vi "VI Tree.vi"   [LabVIEW 2015, in "IT-M3400.lvlib"]
doc: "This is the instrument driver for the <INSTRUMENT NAME>. The VI Tree displays all the user-callable VIs of the instrument driver in an organized table."
uses:
  <instrlib>/IT-M3400/IT-M3400.lvlib
panel:
  # "(c) 2014 <Enter Company Name Here>.  ALL RIGHTS RESERVED."
  # "SEE DIAGRAM\nFOR VI TREE."
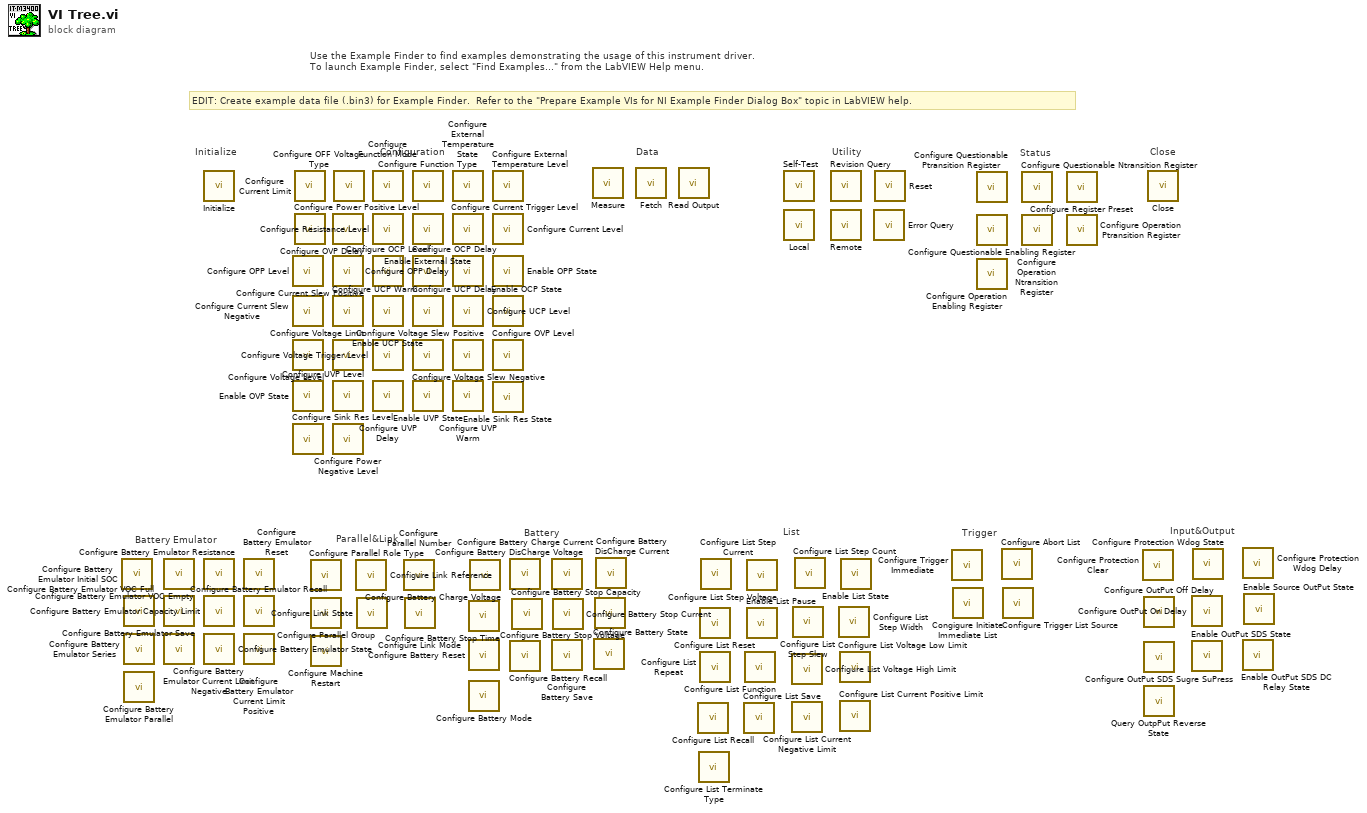
[diagram p0: block diagram]
diagram:
  # "Input&Output"
  # "Trigger"
  # "List"
  # "Battery"
  # "Parallel&Link"
  # "Battery Emulator"
  # "Status"
  # "EDIT: Create example data file (.bin3) for Example Finder.  Refer to the \"Prepare Example VIs for NI Example Finder Dialog Box\" topic in LabVIEW help."
  # "Use the Example Finder to find examples demonstrating the usage of this instrument driver.\nTo launch Example Finder, select \"Find Examples...\" from the LabVIEW Help menu."
  # "Configuration"
  # "Utility"
  # "Data"
  # "Close"
  # "Initialize"
  n1 = call <instrlib>:"Configure Battery Emulator Initial SOC.vi"() -> ()  [unwired: 10 in, 2 out]
  n2 = call <instrlib>:"Configure Battery Emulator VOC Full.vi"() -> ()  [unwired: 10 in, 2 out]
  n3 = call <instrlib>:"Configure Battery Emulator Series.vi"() -> ()  [unwired: 10 in, 2 out]
  n4 = call <instrlib>:"Configure Battery Emulator Parallel.vi"() -> ()  [unwired: 10 in, 2 out]
  n5 = call <instrlib>:"Configure Battery Emulator VOC Empty.vi"() -> ()  [unwired: 10 in, 2 out]
  n6 = call <instrlib>:"Configure Battery Emulator Save.vi"() -> ()  [unwired: 10 in, 2 out]
  n7 = call <instrlib>:"Configure Battery Emulator Current Limit Negative.vi"() -> ()  [unwired: 10 in, 2 out]
  n8 = call <instrlib>:"Initialize.vi"() -> ()  [unwired: 10 in, 2 out]
  n9 = call <instrlib>:"Configure Battery Emulator Resistance.vi"() -> ()  [unwired: 10 in, 2 out]
  n10 = call <instrlib>:"Configure Battery Emulator Capacity Limit.vi"() -> ()  [unwired: 10 in, 2 out]
  n11 = call <instrlib>:"Configure Battery Emulator State.vi"() -> ()  [unwired: 10 in, 2 out]
  n12 = call <instrlib>:"Configure Battery Emulator Reset.vi"() -> ()  [unwired: 10 in, 2 out]
  n13 = call <instrlib>:"Configure Battery Emulator Recall.vi"() -> ()  [unwired: 10 in, 2 out]
  n14 = call <instrlib>:"Configure Battery Emulator Current Limit Positive.vi"() -> ()  [unwired: 10 in, 2 out]
  n15 = call <instrlib>:"Configure OPP Level.vi"() -> ()  [unwired: 10 in, 2 out]
  n16 = call <instrlib>:"Configure Current Slew Negative.vi"() -> ()  [unwired: 10 in, 2 out]
  n17 = call <instrlib>:"Configure Voltage Level.vi"() -> ()  [unwired: 10 in, 2 out]
  n18 = call <instrlib>:"Enable OVP State.vi"() -> ()  [unwired: 10 in, 2 out]
  n19 = call <instrlib>:"Configure Sink Res Level.vi"() -> ()  [unwired: 10 in, 2 out]
  n20 = call <instrlib>:"Configure Current Limit.vi"() -> ()  [unwired: 10 in, 2 out]
  n21 = call <instrlib>:"Configure Power Positive Level.vi"() -> ()  [unwired: 10 in, 2 out]
  n22 = call <instrlib>:"Configure Parallel Role Type.vi"() -> ()  [unwired: 10 in, 2 out]
  n23 = call <instrlib>:"Configure Parallel Group.vi"() -> ()  [unwired: 10 in, 2 out]
  n24 = call <instrlib>:"Configure Machine Restart.vi"() -> ()  [unwired: 10 in, 2 out]
  n25 = call <instrlib>:"Configure OVP Delay.vi"() -> ()  [unwired: 10 in, 2 out]
  n26 = call <instrlib>:"Configure Current Slew Positive.vi"() -> ()  [unwired: 10 in, 2 out]
  n27 = call <instrlib>:"Configure UCP Warm.vi"() -> ()  [unwired: 10 in, 2 out]
  n28 = call <instrlib>:"Configure Voltage Limit.vi"() -> ()  [unwired: 10 in, 2 out]
  n29 = call <instrlib>:"Configure UVP Level.vi"() -> ()  [unwired: 10 in, 2 out]
  n30 = call <instrlib>:"Configure Power Negative Level.vi"() -> ()  [unwired: 10 in, 2 out]
  n31 = call <instrlib>:"Configure OFF Voltage Type.vi"() -> ()  [unwired: 10 in, 2 out]
  n32 = call <instrlib>:"Configure Link Reference.vi"() -> ()  [unwired: 10 in, 2 out]
  n33 = call <instrlib>:"Configure Link State.vi"() -> ()  [unwired: 10 in, 2 out]
  n34 = call <instrlib>:"Configure Function Mode.vi"() -> ()  [unwired: 10 in, 2 out]
  n35 = call <instrlib>:"Configure Resistance Level.vi"() -> ()  [unwired: 10 in, 2 out]
  n36 = call <instrlib>:"Configure OCP Level.vi"() -> ()  [unwired: 10 in, 2 out]
  n37 = call <instrlib>:"Enable UCP State.vi"() -> ()  [unwired: 10 in, 2 out]
  n38 = call <instrlib>:"Configure Voltage Trigger Level.vi"() -> ()  [unwired: 10 in, 2 out]
  n39 = call <instrlib>:"Configure UVP Delay.vi"() -> ()  [unwired: 10 in, 2 out]
  n40 = call <instrlib>:"Configure Parallel Number.vi"() -> ()  [unwired: 10 in, 2 out]
  n41 = call <instrlib>:"Configure Link Mode.vi"() -> ()  [unwired: 10 in, 2 out]
  n42 = call <instrlib>:"Configure Function Type.vi"() -> ()  [unwired: 10 in, 2 out]
  n43 = call <instrlib>:"Enable External State.vi"() -> ()  [unwired: 10 in, 2 out]
  n44 = call <instrlib>:"Configure OCP Delay.vi"() -> ()  [unwired: 10 in, 2 out]
  n45 = call <instrlib>:"Configure UCP Delay.vi"() -> ()  [unwired: 10 in, 2 out]
  n46 = call <instrlib>:"Configure Voltage Slew Negative.vi"() -> ()  [unwired: 10 in, 2 out]
  n47 = call <instrlib>:"Enable UVP State.vi"() -> ()  [unwired: 10 in, 2 out]
  n48 = call <instrlib>:"Configure External Temperature State.vi"() -> ()  [unwired: 10 in, 2 out]
  n49 = call <instrlib>:"Configure Current Trigger Level.vi"() -> ()  [unwired: 10 in, 2 out]
  n50 = call <instrlib>:"Configure OPP Delay.vi"() -> ()  [unwired: 10 in, 2 out]
  n51 = call <instrlib>:"Configure UCP Level.vi"() -> ()  [unwired: 10 in, 2 out]
  n52 = call <instrlib>:"Configure Voltage Slew Positive.vi"() -> ()  [unwired: 10 in, 2 out]
  n53 = call <instrlib>:"Configure UVP Warm.vi"() -> ()  [unwired: 10 in, 2 out]
  n54 = call <instrlib>:"Configure Battery Stop Time.vi"() -> ()  [unwired: 10 in, 2 out]
  n55 = call <instrlib>:"Configure Battery Reset.vi"() -> ()  [unwired: 10 in, 2 out]
  n56 = call <instrlib>:"Configure Battery Mode.vi"() -> ()  [unwired: 10 in, 2 out]
  n57 = call <instrlib>:"Configure Battery Charge Voltage.vi"() -> ()  [unwired: 9 in, 2 out]
  n58 = call <instrlib>:"Configure External Temperature Level.vi"() -> ()  [unwired: 10 in, 2 out]
  n59 = call <instrlib>:"Configure Current Level.vi"() -> ()  [unwired: 10 in, 2 out]
  n60 = call <instrlib>:"Enable OPP State.vi"() -> ()  [unwired: 10 in, 2 out]
  n61 = call <instrlib>:"Enable OCP State.vi"() -> ()  [unwired: 10 in, 2 out]
  n62 = call <instrlib>:"Configure OVP Level.vi"() -> ()  [unwired: 10 in, 2 out]
  n63 = call <instrlib>:"Enable Sink Res State.vi"() -> ()  [unwired: 10 in, 2 out]
  n64 = call <instrlib>:"Configure Battery Charge Current.vi"() -> ()  [unwired: 10 in, 2 out]
  n65 = call <instrlib>:"Configure Battery Recall.vi"() -> ()  [unwired: 10 in, 2 out]
  n66 = call <instrlib>:"Configure Battery Stop Capacity.vi"() -> ()  [unwired: 10 in, 2 out]
  n67 = call <instrlib>:"Configure Battery DisCharge Voltage.vi"() -> ()  [unwired: 10 in, 2 out]
  n68 = call <instrlib>:"Configure Battery Save.vi"() -> ()  [unwired: 10 in, 2 out]
  n69 = call <instrlib>:"Configure Battery Stop Current.vi"() -> ()  [unwired: 10 in, 2 out]
  n70 = call <instrlib>:"Measure.vi"() -> ()  [unwired: 8 in, 3 out]
  n71 = call <instrlib>:"Configure Battery State.vi"() -> ()  [unwired: 10 in, 2 out]
  n72 = call <instrlib>:"Configure Battery Stop Voltage.vi"() -> ()  [unwired: 10 in, 2 out]
  n73 = call <instrlib>:"Configure Battery DisCharge Current.vi"() -> ()  [unwired: 10 in, 2 out]
  n74 = call <instrlib>:"Fetch.vi"() -> ()  [unwired: 9 in, 3 out]
  n75 = call <instrlib>:"Read Output.vi"() -> ()  [unwired: 8 in, 4 out]
  n76 = call <instrlib>:"Configure List Recall.vi"() -> ()  [unwired: 10 in, 2 out]
  n77 = call <instrlib>:"Configure List Terminate Type.vi"() -> ()  [unwired: 9 in, 2 out]
  n78 = call <instrlib>:"Configure List Reset.vi"() -> ()  [unwired: 10 in, 2 out]
  n79 = call <instrlib>:"Configure List Repeat.vi"() -> ()  [unwired: 10 in, 2 out]
  n80 = call <instrlib>:"Configure List Step Current.vi"() -> ()  [unwired: 10 in, 2 out]
  n81 = call <instrlib>:"Configure List Save.vi"() -> ()  [unwired: 10 in, 2 out]
  n82 = call <instrlib>:"Configure List Function.vi"() -> ()  [unwired: 10 in, 2 out]
  n83 = call <instrlib>:"Configure List Step Voltage.vi"() -> ()  [unwired: 10 in, 2 out]
  n84 = call <instrlib>:"Enable List Pause.vi"() -> ()  [unwired: 10 in, 2 out]
  n85 = call <instrlib>:"Self-Test.vi"() -> ()  [unwired: 8 in, 4 out]
  n86 = call <instrlib>:"Local.vi"() -> ()  [unwired: 10 in, 2 out]
  n87 = call <instrlib>:"Configure List Voltage High Limit.vi"() -> ()  [unwired: 10 in, 2 out]
  n88 = call <instrlib>:"Configure List Current Negative Limit.vi"() -> ()  [unwired: 10 in, 2 out]
  n89 = call <instrlib>:"Configure List Step Slew.vi"() -> ()  [unwired: 10 in, 2 out]
  n90 = call <instrlib>:"Configure List Step Count.vi"() -> ()  [unwired: 10 in, 2 out]
  n91 = call <instrlib>:"Revision Query.vi"() -> ()  [unwired: 8 in, 4 out]
  n92 = call <instrlib>:"Remote.vi"() -> ()  [unwired: 10 in, 2 out]
  n93 = call <instrlib>:"Configure List Step Width.vi"() -> ()  [unwired: 10 in, 2 out]
  n94 = call <instrlib>:"Configure List Voltage Low Limit.vi"() -> ()  [unwired: 10 in, 2 out]
  n95 = call <instrlib>:"Configure List Current Positive Limit.vi"() -> ()  [unwired: 10 in, 2 out]
  n96 = call <instrlib>:"Enable List State.vi"() -> ()  [unwired: 10 in, 2 out]
  n97 = call <instrlib>:"Error Query.vi"() -> ()  [unwired: 8 in, 4 out]
  n98 = call <instrlib>:"Reset.vi"() -> ()  [unwired: 10 in, 2 out]
  n99 = call <instrlib>:"Configure Trigger Immediate.vi"() -> ()  [unwired: 10 in, 2 out]
  n100 = call <instrlib>:"Congigure Initiate Immediate List.vi"() -> ()  [unwired: 10 in, 2 out]
  n101 = call <instrlib>:"Configure Questionable Ptransition Register.vi"() -> ()  [unwired: 10 in, 2 out]
  n102 = call <instrlib>:"Configure Questionable Enabling Register.vi"() -> ()  [unwired: 10 in, 2 out]
  n103 = call <instrlib>:"Configure Operation Enabling Register.vi"() -> ()  [unwired: 10 in, 2 out]
  n104 = call <instrlib>:"Configure Abort List.vi"() -> ()  [unwired: 10 in, 2 out]
  n105 = call <instrlib>:"Configure Trigger List Source.vi"() -> ()  [unwired: 10 in, 2 out]
  n106 = call <instrlib>:"Configure Questionable Ntransition Register.vi"() -> ()  [unwired: 10 in, 2 out]
  n107 = call <instrlib>:"Configure Operation Ntransition Register.vi"() -> ()  [unwired: 10 in, 2 out]
  n108 = call <instrlib>:"Configure Register Preset.vi"() -> ()  [unwired: 10 in, 2 out]
  n109 = call <instrlib>:"Configure Operation Ptransition Register.vi"() -> ()  [unwired: 10 in, 2 out]
  n110 = call <instrlib>:"Configure Protection Clear.vi"() -> ()  [unwired: 9 in, 2 out]
  n111 = call <instrlib>:"Configure OutPut Off Delay.vi"() -> ()  [unwired: 10 in, 2 out]
  n112 = call <instrlib>:"Configure OutPut SDS Sugre SuPress.vi"() -> ()  [unwired: 10 in, 2 out]
  n113 = call <instrlib>:"Query OutpPut Reverse State.vi"() -> ()  [unwired: 9 in, 3 out]
  n114 = call <instrlib>:"Close.vi"() -> ()  [unwired: 11 in, 1 out]
  n115 = call <instrlib>:"Configure OutPut On Delay.vi"() -> ()  [unwired: 10 in, 2 out]
  n116 = call <instrlib>:"Enable OutPut SDS State.vi"() -> ()  [unwired: 10 in, 2 out]
  n117 = call <instrlib>:"Configure Protection Wdog State.vi"() -> ()  [unwired: 10 in, 2 out]
  n118 = call <instrlib>:"Configure Protection Wdog Delay.vi"() -> ()  [unwired: 10 in, 2 out]
  n119 = call <instrlib>:"Enable OutPut SDS DC Relay State.vi"() -> ()  [unwired: 10 in, 2 out]
  n120 = call <instrlib>:"Enable Source OutPut State.vi"() -> ()  [unwired: 10 in, 2 out]
